vi "C867_Init.vi"(8 "error in":errorcluster caption="entrée d'erreur") -> (0 "error out":errorcluster caption="sortie d'erreur")   [LabVIEW 2026]
uses:
  C867-VIs/Low Level/PI_GCS2_DLL_x64.dll
panel:
  in  "nBaudRate":i32
  in  "nPortNr":i32
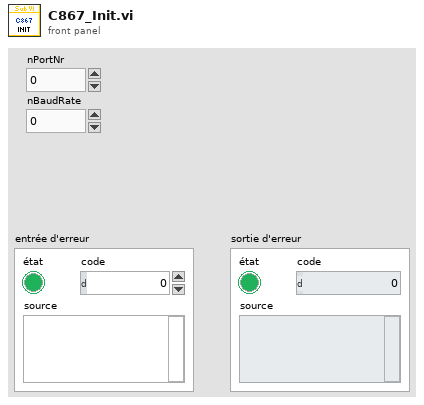
[diagram p1: front panel]
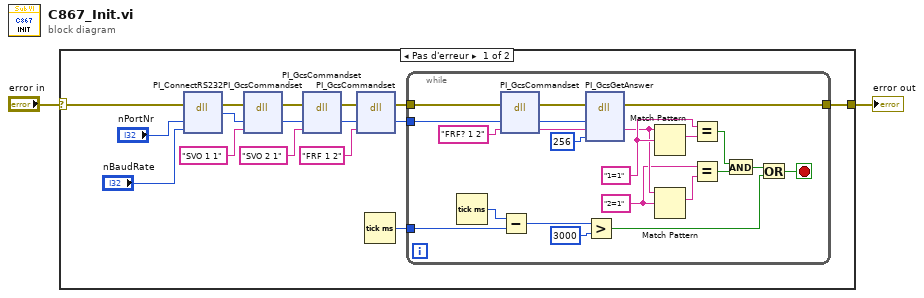
[diagram p0: block diagram]
diagram:
  n1 = case shown="Pas d'erreur" "error in" {
    selector: "error in" -> [w18 w41]
    tunnel: [w4 w41] -> w1
    frame No Error {
      n2 = dll-call lib="C:/Users/Sebastien/Documents/GitHub/LABVIEW-Useful-codes/Device_control/PC-C867-IO Control/v0.1/SubVI/PI-C867/C867-VIs/Low Level/PI_GCS2_DLL_x64.dll" fn="PI_ConnectRS232"(error in=w18, "nPortNr"="nPortNr", "nBaudRate"="nBaudRate") -> (error out=w17:errorcluster, "ID"=w14:i32)  [unwired: 4 in, 1 out]
      n3 = dll-call lib="C:/Users/Sebastien/Documents/GitHub/LABVIEW-Useful-codes/Device_control/PC-C867-IO Control/v0.1/SubVI/PI-C867/C867-VIs/Low Level/PI_GCS2_DLL_x64.dll" fn="PI_GcsCommandset"(error in=w17, "ID"=w14, "szCommand"="SVO 1 1") -> (error out=w12:errorcluster, "ID"=w11:i32)  [unwired: 4 in, 1 out]
      n4 = dll-call lib="C:/Users/Sebastien/Documents/GitHub/LABVIEW-Useful-codes/Device_control/PC-C867-IO Control/v0.1/SubVI/PI-C867/C867-VIs/Low Level/PI_GCS2_DLL_x64.dll" fn="PI_GcsCommandset"(error in=w12, "ID"=w11, "szCommand"="SVO 2 1") -> (error out=w9:errorcluster, "ID"=w8:i32)  [unwired: 4 in, 1 out]
      n5 = dll-call lib="C:/Users/Sebastien/Documents/GitHub/LABVIEW-Useful-codes/Device_control/PC-C867-IO Control/v0.1/SubVI/PI-C867/C867-VIs/Low Level/PI_GCS2_DLL_x64.dll" fn="PI_GcsCommandset"(error in=w9, "ID"=w8, "szCommand"="FRF 1 2") -> (error out=w6:errorcluster, "ID"=w5:i32)  [unwired: 4 in, 1 out]
      n6 = Tick Count (ms)() -> (millisecond timer value=w3:u32)
      n7 = while {
        tunnel: w6 -> [w40]
        tunnel: w5 -> [w39]
        tunnel: [w36] -> w4
        tunnel: w3 -> [w31]
        stop <- w19 stop-if-true
        w24 = "2=1" ("chaîne recherchée")
        w28 = "1=1" ("chaîne recherchée")
        n8 = Tick Count (ms)() -> (millisecond timer value=w32:u32)
        n9 = dll-call lib="C:/Users/Sebastien/Documents/GitHub/LABVIEW-Useful-codes/Device_control/PC-C867-IO Control/v0.1/SubVI/PI-C867/C867-VIs/Low Level/PI_GCS2_DLL_x64.dll" fn="PI_GcsCommandset"(error in=w40, "ID"=w39, "szCommand"="FRF? 1 2") -> (error out=w37:errorcluster, "ID"=w35:i32, "szCommand"=w33:string)  [unwired: 3 in, 1 out]
        n10 = Subtract(x=w32, y=w31) -> (x-y=w30:u32)
        n11 = dll-call lib="C:/Users/Sebastien/Documents/GitHub/LABVIEW-Useful-codes/Device_control/PC-C867-IO Control/v0.1/SubVI/PI-C867/C867-VIs/Low Level/PI_GCS2_DLL_x64.dll" fn="PI_GcsGetAnswer"(error in=w37, "ID"=w35, "buffer"=w33, "buffersize"=256) -> (error out=w36:errorcluster, "buffer"=w26:string)  [unwired: 5 in, 1 out]
        n12 = Greater?(x=w30, y=u32 3000) -> (0:w20:bool)
        n13 = Match Pattern(string=w26, regular expression=w28) -> (match substring=w27:string)  [unwired: 1 in, 3 out]
        n14 = Match Pattern(string=w26, regular expression=w24) -> (match substring=w25:string)  [unwired: 1 in, 3 out]
        n15 = Equal?(x=w28, y=w27) -> (x = y?=w23:bool)
        n16 = Equal?(x=w24, y=w25) -> (x = y?=w22:bool)
        n17 = And(x=w23, y=w22) -> (x .and. y?=w21:bool)
        n18 = Or(x=w21, y=w20) -> (x .or. y?=w19:bool)
      }
    }
    frame Error {
    }
  }
  "error out" <- w1
